vi "Save Settings To DB.vi"(6 "Save To File?":bool, 7 "Dashboard?":bool, 8 "error in":errorcluster, 9 "Drive PID - High":T1, 10 "save file (in)":T2, 11 "Drive PID - Low":T1) -> (0 "error out":errorcluster, 2 "save file (out)":T2)   [LabVIEW 2016]
uses:
  PID Settings.ctl
  <vilib>/Utility/config.llb/Config Data RefNum.ctl
  Load Save Info.ctl
  <vilib>/Utility/config.llb/NI_LVConfig.lvlib
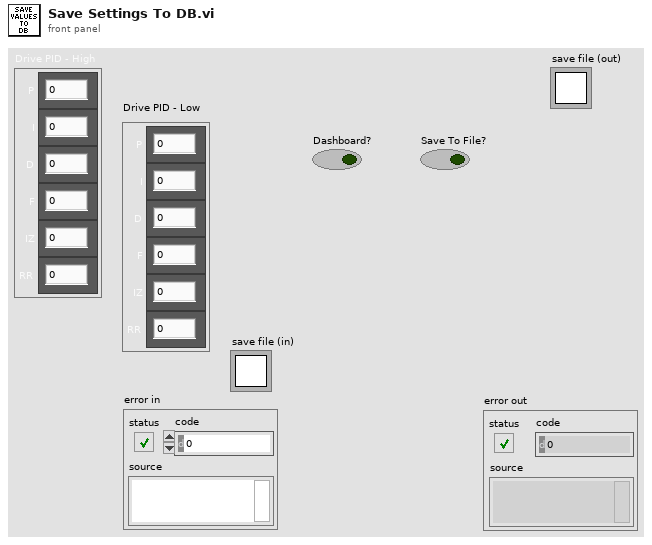
[diagram p1: front panel]
types:
  T1 = typedef "PID Settings.ctl" = cluster{"D":dbl, "F":dbl, "RR":dbl, "IZ":dbl, "P":dbl, "I":dbl}
  T2 = typedef "NI_LVConfig.lvlib/Config Data RefNum.ctl" = refnum<k1>
  T3 = typedef "Load Save Info.ctl" = cluster{"Load?":bool, "Dashboard?":bool, "save file":T2, "File?":bool}
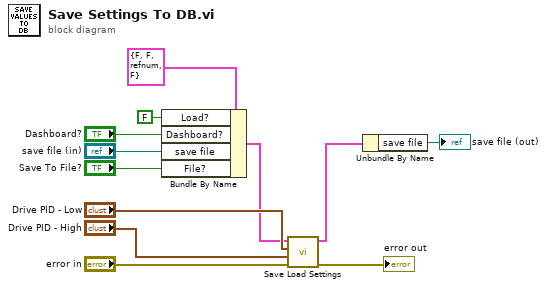
[diagram p0: block diagram]
diagram:
  n1 = Bundle By Name(cluster=T3 {"Load?"=FALSE, "Dashboard?"=FALSE, "save file"=refnum, "File?"=FALSE} ("Save Load Info"), "Load?"=FALSE, "Dashboard?"="Dashboard?", "save file"="save file (in)", "File?"="Save To File?") -> (w8:T3)
  n2 = call "Save Load Settings.vi"("error in"="error in", "Drive PID - High (in)"="Drive PID - High", "Drive PID - Low (in)"="Drive PID - Low", "Save Load Info"=w8) -> ("error out"=→"error out":errorcluster, "Save Load Info (out)"=w3:T3)  [unwired: 4 in, 2 out]
  n3 = Unbundle By Name(w3) -> ("save file"=→"save file (out)":T2)
